vi "Configure Marker Search.vi"(0 "VISA resource name":refnum<visa-resource-name>, 1 "Peak Excursion (6 dB)":dbl=6.0, 2 "Peak Threshold (-90 dBm)":dbl=-90.0, 3 "Peak Search Type (0: Maximum Value)":u16(ring) items=["Maximum Value", "Excursion And Threshold"], 5 "Active Marker (1: Marker1)":u16(ring)=1 items=["Marker1"=1, "Marker2"=2, "Marker3"=3, "Marker4"=4], 7 "Enable Auto N dB Points (T: Enable)":bool=TRUE, 9 "Manual N dB Points (-3 dB)":i32=-3, 11 "error in (no error)":errorcluster) -> (4 "VISA resource name out":refnum<visa-resource-name>, 15 "error out":errorcluster)   [LabVIEW 2014, in "Agilent ESA PSA Series.lvlib"]
doc: "Configures the marker search."
uses:
  Agilent ESA PSA Series.lvlib
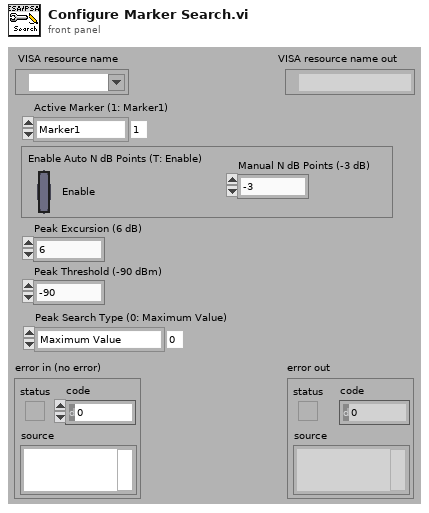
[diagram p1: front panel]
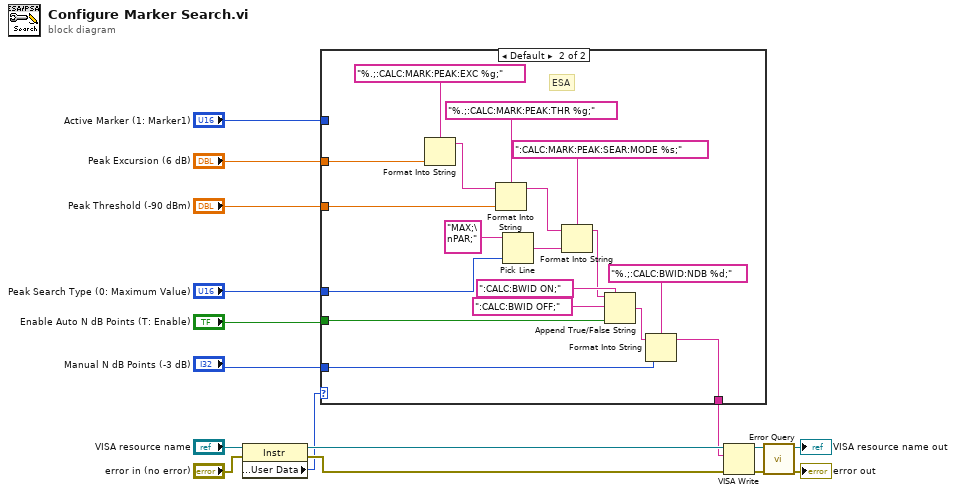
[diagram p0: block diagram]
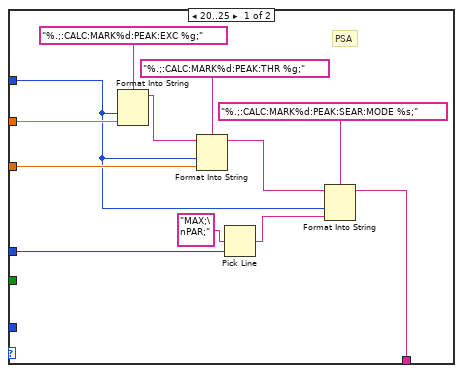
[diagram p2: hidden frame]
diagram:
  n1 = property on="Property Node" class="Instr"(reference="VISA resource name", error in="error in (no error)") -> (reference out=w10:refnum<visa-resource-name>, error out=w9:errorcluster, "General Settings:User Data"=w8:u32)
  n2 = case shown="Default" w8 {
    tunnel: "Enable Auto N dB Points (T: Enable)" -> [_ w46]
    tunnel: [w20 w42] -> w6
    tunnel: "Manual N dB Points (-3 dB)" -> [_ w41]
    tunnel: "Peak Search Type (0: Maximum Value)" -> [w22 w40]
    tunnel: "Peak Excursion (6 dB)" -> [w19 w39]
    tunnel: "Peak Threshold (-90 dBm)" -> [w18 w34]
    tunnel: "Active Marker (1: Marker1)" -> [w17 _]
    frame 20..25 {
      # "PSA"
      n3 = Format Into String(format string="%.;:CALC:MARK%d:PEAK:EXC %g;", w17, w19) -> (resulting string=w25:string)  [unwired: 2 in, 1 out]
      n4 = Format Into String(format string="%.;:CALC:MARK%d:PEAK:THR %g;", initial string=w25, w17, w18) -> (resulting string=w27:string)  [unwired: 1 in, 1 out]
      n5 = Pick Line(multi-line string="MAX;\nPAR;", line index=w22) -> (output string=w21:string)  [unwired: 1 in]
      n6 = Format Into String(format string="%.;:CALC:MARK%d:PEAK:SEAR:MODE %s;", initial string=w27, w17, w21) -> (resulting string=w20:string)  [unwired: 1 in, 1 out]
    }
    frame Default {
      # "ESA"
      n7 = Format Into String(format string="%.;:CALC:MARK:PEAK:EXC %g;", w39) -> (resulting string=w36:string)  [unwired: 2 in, 1 out]
      n8 = Format Into String(format string="%.;:CALC:MARK:PEAK:THR %g;", initial string=w36, w34) -> (resulting string=w32:string)  [unwired: 1 in, 1 out]
      n9 = Pick Line(multi-line string="MAX;\nPAR;", line index=w40) -> (output string=w31:string)  [unwired: 1 in]
      n10 = Format Into String(format string=":CALC:MARK:PEAK:SEAR:MODE %s;", initial string=w32, w31) -> (resulting string=w29:string)  [unwired: 1 in, 1 out]
      n11 = Append True/False String(1:w46, 2:":CALC:BWID OFF;" ("true string"), 3:":CALC:BWID ON;" ("true string"), 4:w29) -> (0:w43:string)
      n12 = Format Into String(format string="%.;:CALC:BWID:NDB %d;", initial string=w43, w41) -> (resulting string=w42:string)  [unwired: 1 in, 1 out]
    }
  }
  n13 = VISA Write(VISA resource name=w10, write buffer=w6, error in (no error)=w9) -> (VISA resource name out=w16:refnum<visa-resource-name>, error out=w14:errorcluster)  [unwired: 1 out]
  n14 = call "Error Query.vi"("error in (no error)"=w14, "VISA resource name"=w16) -> ("error out"=→"error out":errorcluster, "VISA resource name out"=→"VISA resource name out":refnum<visa-resource-name>)  [unwired: 6 in, 2 out]
